vi "Measure [MSR].vi"(8 "error in (no error)":errorcluster, 9 "measurement type (voltage)":i32(ring)=1 items=["Voltage"=1, "Current"=0], 10 "channel name (\"CHANNEL1\")":string="CHANNEL1", 11 "Cs++DCPwr in":refnum<class "CS++DCPwr.lvclass">) -> (0 "error out":errorcluster, 2 "measurement":dbl format="%^.2e", 3 "CS++DCPwr out":refnum<class "CS++DCPwr.lvclass">)   [LabVIEW 2015, in "CS++DCPwr.lvlib" / "CS++DCPwr.lvclass"]
doc: "This VI takes a single measurement on the channel you specify.\n\nNotes:\n\n(1) This VI is part of the IviDCPwrMeasure [MSR] extension group."
uses:
  CS++DCPwr.lvclass
  CS++DCPwr.lvclass/CS++DCPwr.ctl
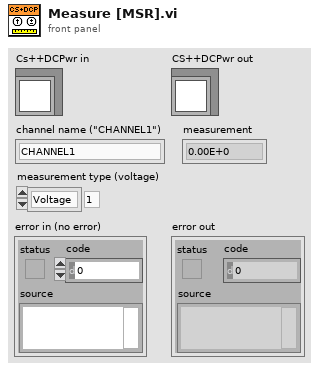
[diagram p1: front panel]
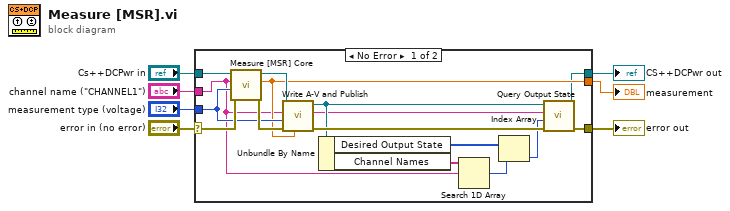
[diagram p0: block diagram]
diagram:
  n1 = case shown="No Error" "error in (no error)" {
    selector: "error in (no error)" -> [w21 w24]
    tunnel: [w14 w24] -> w6
    tunnel: [w16 w23] -> w4
    tunnel: "Cs++DCPwr in" -> [w22 w23]
    tunnel: "channel name (\"CHANNEL1\")" -> [w11 _]
    tunnel: "measurement type (voltage)" -> [w18 _]
    tunnel: [w17 _] -> w1
    frame No Error {
      n2 = call-dynamic "Measure [MSR] Core.vi"("error in (no error)"=w21, "measurement type (voltage)"=w18, "channel name (\"CHANNEL1\")"=w11, "Cs++DCPwr in"=w22) -> ("error out"=w19:errorcluster, "measurement"=w17:dbl, "CS++DCPwr out"=w20:refnum<class "CS++DCPwr.lvclass">)  [unwired: 5 in]
      n3 = call "Write A-V and Publish.vi"("measurement"=w17, "error in (no error)"=w19, "measurement type (voltage)"=w18, "channel name (\"CHANNEL1\")"=w11, "CS++DCPwr in"=w20) -> ("error out"=w15:errorcluster, "CS++DCPwr out"=w13:refnum<class "CS++DCPwr.lvclass">)  [unwired: 5 in]
      n4 = Unbundle By Name(w13) -> ("Desired Output State"=w10:i32[], "Channel Names"=w12:string[])
      n5 = Search 1D Array(1D array=w12, element=w11) -> (index of element=w9:i32)  [unwired: 1 in]
      n6 = Index Array(array=w10, index=w9) -> (element=w8:i32)
      n7 = call "Query Output State.vi"("error in (no error)"=w15, "output state (Constant Voltage)"=w8, "channel name (\"CHANNEL1\")"=w11, "CS++DCPwr in"=w13) -> ("error out"=w14:errorcluster, "CS++DCPwr out"=w16:refnum<class "CS++DCPwr.lvclass">)  [unwired: 5 in, 1 out]
    }
    frame Error {
    }
  }
  "error out" <- w6
  "CS++DCPwr out" <- w4
  "measurement" <- w1
